vi "REV2mDistanceSensor Set Profile.vi"(10 "Profile":T1, 11 "REV2mDistanceSensorDevRef":T2) -> (3 "REV2mDistanceSensorDevRef Out":T2)   [LabVIEW 2019, in "DistanceSensorDriver.lvlib"]
uses:
  DistanceSensorDriver.lvlib
  Typedef/REV2mDistanceSensorDevRef.ctl
  Typedef/Ports.ctl
  Typedef/RangeProfile.ctl
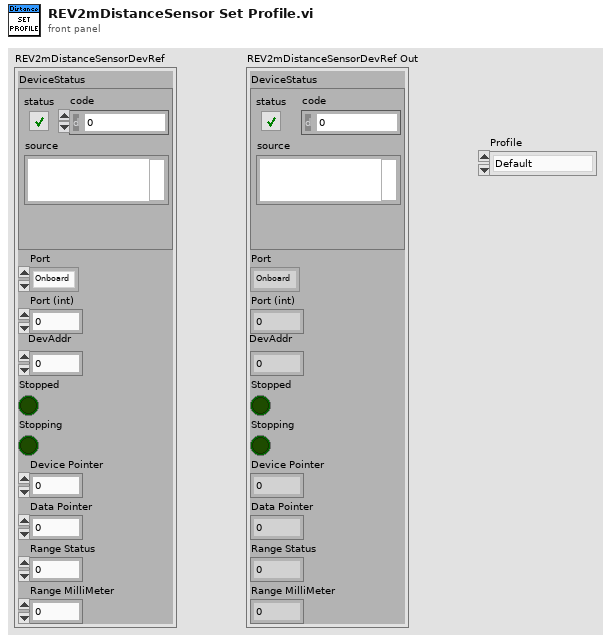
[diagram p1: front panel]
types:
  T1 = typedef "DistanceSensorDriver.lvlib/RangeProfile.ctl" = enum16{"Default", "High Speed", "High Accuracy", "Long Range"}
  T2 = typedef "DistanceSensorDriver.lvlib/REV2mDistanceSensorDevRef.ctl" = cluster{"DeviceStatus":errorcluster, "Port":T3, "Port (int)":i32, "DevAddr":i32, "Stopped":bool, "Stopping":bool, "Device Pointer":u64, "Data Pointer":u64, "Range Status":u8, "Range MilliMeter":u16}
  T3 = typedef "DistanceSensorDriver.lvlib/Ports.ctl" = enum32{"Onboard", "MXP"}
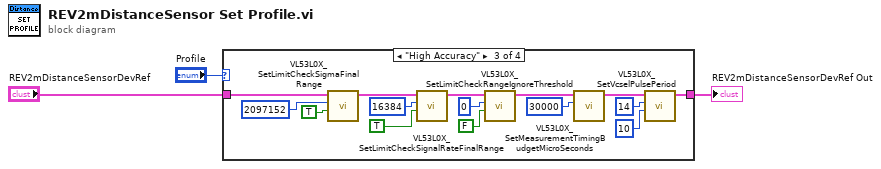
[diagram p0: block diagram]
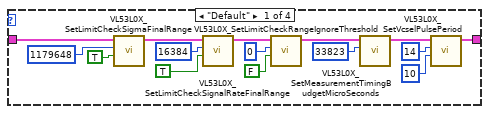
[diagram p2: hidden frame]
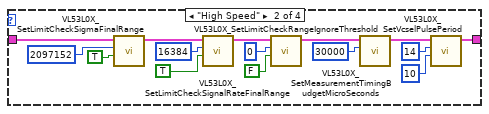
[diagram p3: hidden frame]
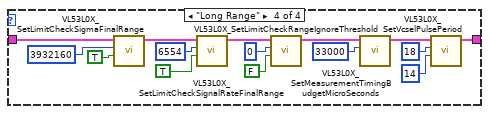
[diagram p4: hidden frame]
diagram:
  n1 = case shown="\"High Accuracy\"" "Profile" {
    tunnel: "REV2mDistanceSensorDevRef" -> [w5 w20 w35 w56]
    tunnel: [w4 w19 w34 w55] -> w1
    frame "Default" {
      n2 = call "VL53L0X_SetLimitCheckSigmaFinalRange.vi"("Enable (T)"=TRUE, "LimitCheckValue"=u32 1179648 ("value"), "REV2mDistanceSensorDevRef"=w5) -> ("REV2mDistanceSensorDevRef Out"=w15:T2)  [unwired: 8 in]
      n3 = call "VL53L0X_SetLimitCheckSignalRateFinalRange.vi"("Enable (T)"=TRUE, "LimitCheckValue"=u32 16384, "REV2mDistanceSensorDevRef"=w15) -> ("REV2mDistanceSensorDevRef Out"=w16:T2)  [unwired: 8 in]
      n4 = call "VL53L0X_SetLimitCheckRangeIgnoreThreshold.vi"("Enable (T)"=FALSE, "LimitCheckValue"=u32 0, "REV2mDistanceSensorDevRef"=w16) -> ("REV2mDistanceSensorDevRef Out"=w17:T2)  [unwired: 8 in]
      n5 = call "VL53L0X_SetMeasurementTimingBudgetMicroSeconds.vi"("MeasurementTimingBudgetMicroSeconds"=u32 33823 ("val"), "REV2mDistanceSensorDevRef"=w17) -> ("REV2mDistanceSensorDevRef Out"=w18:T2)  [unwired: 9 in]
      n6 = call "VL53L0X_SetVcselPulsePeriod.vi"("VCSELPulsePeriodPCLK Final"=u8 10 ("Final Range"), "VCSELPulsePeriodPCLK Pre"=u8 14 ("Pre Range"), "REV2mDistanceSensorDevRef"=w18) -> ("REV2mDistanceSensorDevRef Out"=w4:T2)  [unwired: 8 in]
    }
    frame "High Speed" {
      n7 = call "VL53L0X_SetLimitCheckSigmaFinalRange.vi"("Enable (T)"=TRUE, "LimitCheckValue"=u32 2097152 ("value"), "REV2mDistanceSensorDevRef"=w20) -> ("REV2mDistanceSensorDevRef Out"=w30:T2)  [unwired: 8 in]
      n8 = call "VL53L0X_SetLimitCheckSignalRateFinalRange.vi"("Enable (T)"=TRUE, "LimitCheckValue"=u32 16384, "REV2mDistanceSensorDevRef"=w30) -> ("REV2mDistanceSensorDevRef Out"=w31:T2)  [unwired: 8 in]
      n9 = call "VL53L0X_SetLimitCheckRangeIgnoreThreshold.vi"("Enable (T)"=FALSE, "LimitCheckValue"=u32 0, "REV2mDistanceSensorDevRef"=w31) -> ("REV2mDistanceSensorDevRef Out"=w32:T2)  [unwired: 8 in]
      n10 = call "VL53L0X_SetMeasurementTimingBudgetMicroSeconds.vi"("MeasurementTimingBudgetMicroSeconds"=u32 30000 ("val"), "REV2mDistanceSensorDevRef"=w32) -> ("REV2mDistanceSensorDevRef Out"=w33:T2)  [unwired: 9 in]
      n11 = call "VL53L0X_SetVcselPulsePeriod.vi"("VCSELPulsePeriodPCLK Final"=u8 10 ("Final Range"), "VCSELPulsePeriodPCLK Pre"=u8 14 ("Pre Range"), "REV2mDistanceSensorDevRef"=w33) -> ("REV2mDistanceSensorDevRef Out"=w19:T2)  [unwired: 8 in]
    }
    frame "High Accuracy" {
      n12 = call "VL53L0X_SetLimitCheckSigmaFinalRange.vi"("Enable (T)"=TRUE, "LimitCheckValue"=u32 2097152 ("value"), "REV2mDistanceSensorDevRef"=w35) -> ("REV2mDistanceSensorDevRef Out"=w48:T2)  [unwired: 8 in]
      n13 = call "VL53L0X_SetLimitCheckSignalRateFinalRange.vi"("Enable (T)"=TRUE, "LimitCheckValue"=u32 16384, "REV2mDistanceSensorDevRef"=w48) -> ("REV2mDistanceSensorDevRef Out"=w47:T2)  [unwired: 8 in]
      n14 = call "VL53L0X_SetLimitCheckRangeIgnoreThreshold.vi"("Enable (T)"=FALSE, "LimitCheckValue"=u32 0, "REV2mDistanceSensorDevRef"=w47) -> ("REV2mDistanceSensorDevRef Out"=w46:T2)  [unwired: 8 in]
      n15 = call "VL53L0X_SetMeasurementTimingBudgetMicroSeconds.vi"("MeasurementTimingBudgetMicroSeconds"=u32 30000 ("val"), "REV2mDistanceSensorDevRef"=w46) -> ("REV2mDistanceSensorDevRef Out"=w45:T2)  [unwired: 9 in]
      n16 = call "VL53L0X_SetVcselPulsePeriod.vi"("VCSELPulsePeriodPCLK Final"=u8 10 ("Final Range"), "VCSELPulsePeriodPCLK Pre"=u8 14 ("Pre Range"), "REV2mDistanceSensorDevRef"=w45) -> ("REV2mDistanceSensorDevRef Out"=w34:T2)  [unwired: 8 in]
    }
    frame "Long Range" {
      n17 = call "VL53L0X_SetLimitCheckSigmaFinalRange.vi"("Enable (T)"=TRUE, "LimitCheckValue"=u32 3932160 ("value"), "REV2mDistanceSensorDevRef"=w56) -> ("REV2mDistanceSensorDevRef Out"=w60:T2)  [unwired: 8 in]
      n18 = call "VL53L0X_SetLimitCheckSignalRateFinalRange.vi"("Enable (T)"=TRUE, "LimitCheckValue"=u32 6554, "REV2mDistanceSensorDevRef"=w60) -> ("REV2mDistanceSensorDevRef Out"=w61:T2)  [unwired: 8 in]
      n19 = call "VL53L0X_SetLimitCheckRangeIgnoreThreshold.vi"("Enable (T)"=FALSE, "LimitCheckValue"=u32 0, "REV2mDistanceSensorDevRef"=w61) -> ("REV2mDistanceSensorDevRef Out"=w62:T2)  [unwired: 8 in]
      n20 = call "VL53L0X_SetMeasurementTimingBudgetMicroSeconds.vi"("MeasurementTimingBudgetMicroSeconds"=u32 33000 ("val"), "REV2mDistanceSensorDevRef"=w62) -> ("REV2mDistanceSensorDevRef Out"=w63:T2)  [unwired: 9 in]
      n21 = call "VL53L0X_SetVcselPulsePeriod.vi"("VCSELPulsePeriodPCLK Final"=u8 14 ("Final Range"), "VCSELPulsePeriodPCLK Pre"=u8 18 ("Pre Range"), "REV2mDistanceSensorDevRef"=w63) -> ("REV2mDistanceSensorDevRef Out"=w55:T2)  [unwired: 8 in]
    }
  }
  "REV2mDistanceSensorDevRef Out" <- w1
